vi "MainFormulas.vi"() -> ()   [LabVIEW 2020]
doc: "Zawiera podstawowe wzory matematyczne i fizyczne, Demonstrator na potrzeby kursu LabVIEW."
panel:
  in  "MainTab":enum32{"FIZYCZNE", "MATEMATYCZNE"}(tab)
  in  "Math":T1(tab)
  in  "R_eq_button":bool
  in  "R":dbl[](array[numeric]) caption="R [Ohm]"
  in  "Connect":enum16{"SZEREGOWO", "RÓWNOLEGLE"}(ring) caption="Rodzaj połączenia"
  out "R_eq":dbl caption="R_Z [Ohm]" format="%#.2g"
  in  "C_eq_button":bool
  in  "C":dbl[](array[numeric])
  in  "Connect 2":enum16{"SZEREGOWO", "RÓWNOLEGLE"}(ring) caption="Rodzaj połączenia"
  out "C_eq":dbl caption="C_Z  [Farad]" format="%#.2g"
  in  "Physics":enum32{"POLA FIGUR", "PITAGORAS"}(tab)
  # "R=R1+R2"
  # "1/R=1/R1+1/R2"
  # "C=1/C1+1/C2"
  # "C=C1+C2"
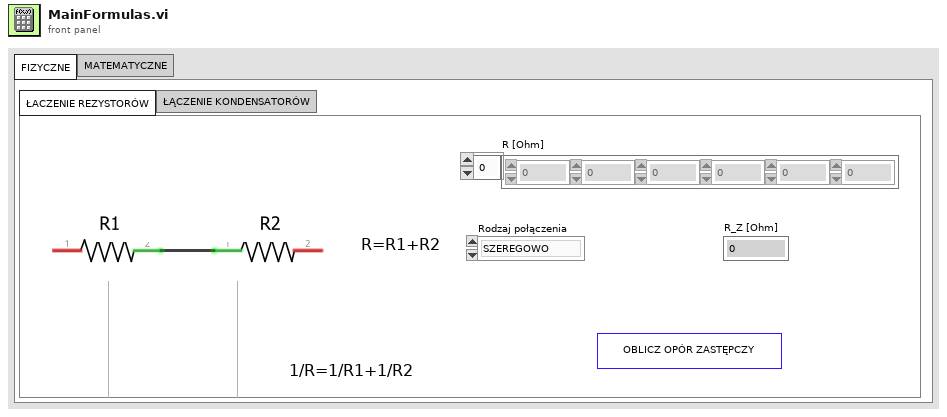
[diagram p1: front panel]
types:
  T1 = enum32{"ŁACZENIE REZYSTORÓW", "ŁĄCZENIE KONDENSATORÓW"}
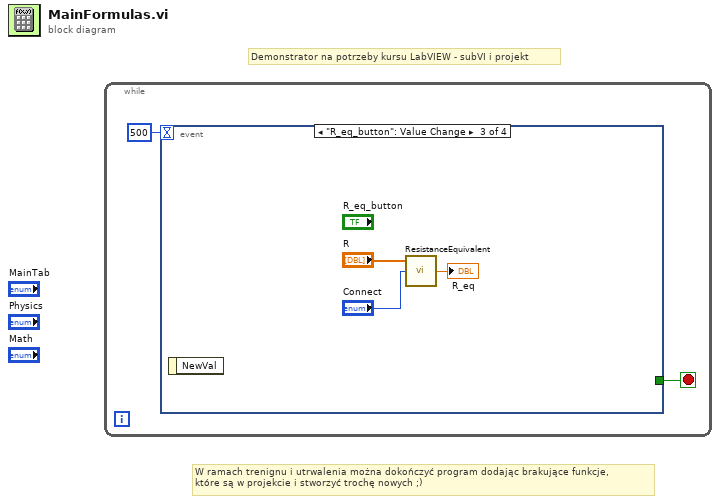
[diagram p0: block diagram]
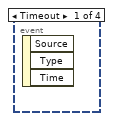
[diagram p2: hidden frame]
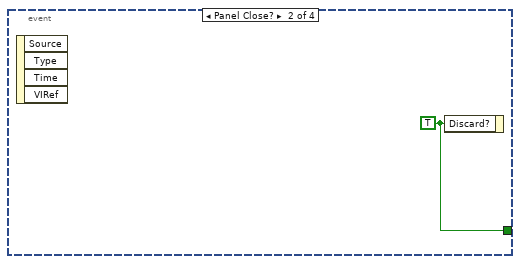
[diagram p3: hidden frame]
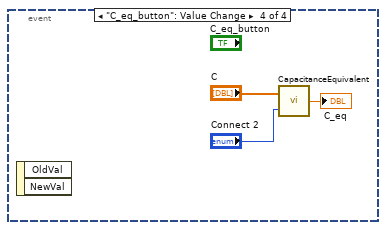
[diagram p4: hidden frame]
diagram:
  # "W ramach trenignu i utrwalenia można dokończyć program dodając brakujące funkcje,\nktóre są w projekcie i stworzyć trochę nowych ;)"
  # "Demonstrator na potrzeby kursu LabVIEW - subVI i projekt"
  n1 = while {
    stop <- w1 stop-if-true
    n2 = event shown="[2] \"R_eq_button\": Value Change" {
      selector: _ -> [_ _ _ _]
      dyn-events: _ -> [_ _ _ _]
      timeout: 500 -> [_ _ _ _]
      tunnel: [_ w3 _ _] -> w1
      event Timeout {
        n3 = event-data() -> ()  [unwired: 1 in, 3 out]
      }
      event Panel Close? {
        w3 = TRUE ("Discard?")
        n4 = event-data() -> ()  [unwired: 1 in, 4 out]
        n5 = event-data("Discard?"=w3) -> ()  [unwired: 1 in, 1 out]
      }
      event "R_eq_button": Value Change {
        n6 = event-data() -> ()  [unwired: 1 in, 1 out]
        n7 = call "ResistanceEquivalent.vi"("Connect"="Connect", "R"="R") -> ("R_eq"=→"R_eq":dbl)  [unwired: 2 in]
      }
      event "C_eq_button": Value Change {
        n8 = event-data() -> ()  [unwired: 1 in, 2 out]
        n9 = call "CapacitanceEquivalent.vi"("Connect"="Connect 2", "C"="C") -> ("C_eq"=→"C_eq":dbl)
      }
    }
  }
